vi "Empty Array__ogtk.vi"   [LabVIEW 2012]
doc: "Returns TRUE if Array is empty (any dimension has length equal zero). Otherwise, this function returns FALSE."
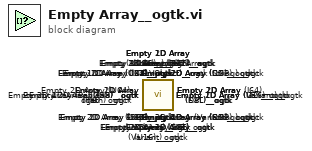
[diagram p0: block diagram]
diagram:
  n1 = call <userlib>:"Empty 2D Array (LVObject)__ogtk.vi"() -> ()  [unwired: 9 in, 1 out]
  n2 = call <userlib>:"Empty 1D Array (LVObject)__ogtk.vi"() -> ()  [unwired: 9 in, 1 out]
  n3 = call <userlib>:"Empty 2D Array (U64)__ogtk.vi"() -> ()  [unwired: 9 in, 1 out]
  n4 = call <userlib>:"Empty 2D Array (I64)__ogtk.vi"() -> ()  [unwired: 9 in, 1 out]
  n5 = call <userlib>:"Empty 1D Array (U64)__ogtk.vi"() -> ()  [unwired: 9 in, 1 out]
  n6 = call <userlib>:"Empty 1D Array (I64)__ogtk.vi"() -> ()  [unwired: 9 in, 1 out]
  n7 = call <userlib>:"Empty Array (Variant)__ogtk.vi"() -> ()  [unwired: 9 in, 1 out]
  n8 = call <userlib>:"Empty 2D Array (Variant)__ogtk.vi"() -> ()  [unwired: 9 in, 1 out]
  n9 = call <userlib>:"Empty 2D Array (U32)__ogtk.vi"() -> ()  [unwired: 9 in, 1 out]
  n10 = call <userlib>:"Empty 2D Array (U16)__ogtk.vi"() -> ()  [unwired: 9 in, 1 out]
  n11 = call <userlib>:"Empty 2D Array (U8)__ogtk.vi"() -> ()  [unwired: 9 in, 1 out]
  n12 = call <userlib>:"Empty 2D Array (String)__ogtk.vi"() -> ()  [unwired: 9 in, 1 out]
  n13 = call <userlib>:"Empty 2D Array (SGL)__ogtk.vi"() -> ()  [unwired: 9 in, 1 out]
  n14 = call <userlib>:"Empty 2D Array (Path)__ogtk.vi"() -> ()  [unwired: 9 in, 1 out]
  n15 = call <userlib>:"Empty 2D Array (I32)__ogtk.vi"() -> ()  [unwired: 9 in, 1 out]
  n16 = call <userlib>:"Empty 2D Array (I16)__ogtk.vi"() -> ()  [unwired: 9 in, 1 out]
  n17 = call <userlib>:"Empty 2D Array (I8)__ogtk.vi"() -> ()  [unwired: 9 in, 1 out]
  n18 = call <userlib>:"Empty 2D Array (EXT)__ogtk.vi"() -> ()  [unwired: 9 in, 1 out]
  n19 = call <userlib>:"Empty 2D Array (DBL)__ogtk.vi"() -> ()  [unwired: 9 in, 1 out]
  n20 = call <userlib>:"Empty 2D Array (CSG)__ogtk.vi"() -> ()  [unwired: 9 in, 1 out]
  n21 = call <userlib>:"Empty 2D Array (CXT)__ogtk.vi"() -> ()  [unwired: 9 in, 1 out]
  n22 = call <userlib>:"Empty 2D Array (CDB)__ogtk.vi"() -> ()  [unwired: 9 in, 1 out]
  n23 = call <userlib>:"Empty 2D Array (Boolean)__ogtk.vi"() -> ()  [unwired: 9 in, 1 out]
  n24 = call <userlib>:"Empty 1D Array (Variant)__ogtk.vi"() -> ()  [unwired: 9 in, 1 out]
  n25 = call <userlib>:"Empty 1D Array (U32)__ogtk.vi"() -> ()  [unwired: 9 in, 1 out]
  n26 = call <userlib>:"Empty 1D Array (U16)__ogtk.vi"() -> ()  [unwired: 9 in, 1 out]
  n27 = call <userlib>:"Empty 1D Array (U8)__ogtk.vi"() -> ()  [unwired: 9 in, 1 out]
  n28 = call <userlib>:"Empty 1D Array (String)__ogtk.vi"() -> ()  [unwired: 9 in, 1 out]
  n29 = call <userlib>:"Empty 1D Array (SGL)__ogtk.vi"() -> ()  [unwired: 9 in, 1 out]
  n30 = call <userlib>:"Empty 1D Array (Path)__ogtk.vi"() -> ()  [unwired: 9 in, 1 out]
  n31 = call <userlib>:"Empty 1D Array (I32)__ogtk.vi"() -> ()  [unwired: 9 in, 1 out]
  n32 = call <userlib>:"Empty 1D Array (I16)__ogtk.vi"() -> ()  [unwired: 9 in, 1 out]
  n33 = call <userlib>:"Empty 1D Array (I8)__ogtk.vi"() -> ()  [unwired: 9 in, 1 out]
  n34 = call <userlib>:"Empty 1D Array (EXT)__ogtk.vi"() -> ()  [unwired: 9 in, 1 out]
  n35 = call <userlib>:"Empty 1D Array (DBL)__ogtk.vi"() -> ()  [unwired: 9 in, 1 out]
  n36 = call <userlib>:"Empty 1D Array (CSG)__ogtk.vi"() -> ()  [unwired: 9 in, 1 out]
  n37 = call <userlib>:"Empty 1D Array (CXT)__ogtk.vi"() -> ()  [unwired: 9 in, 1 out]
  n38 = call <userlib>:"Empty 1D Array (CDB)__ogtk.vi"() -> ()  [unwired: 9 in, 1 out]
  n39 = call <userlib>:"Empty 1D Array (Boolean)__ogtk.vi"() -> ()  [unwired: 9 in, 1 out]
